vi "WriteLog.vi"(8 "error in (no error)":errorcluster, 10 "Loop Counter":i32, 11 "Channel Manager in":refnum<class "Channel Manager.lvclass">) -> (0 "error out":errorcluster, 3 "Channel Manager out":refnum<class "Channel Manager.lvclass">)   [LabVIEW 2024, in "Embedded TDMS Logger Engine.lvlib" / "Channel Manager.lvclass"]
doc: "Write to our TDMS file if the trigger is active."
uses:
  Channel Manager.lvclass
  Channel Manager.lvclass/Channel Manager.ctl
  Shared/File Classes/File/File.lvclass
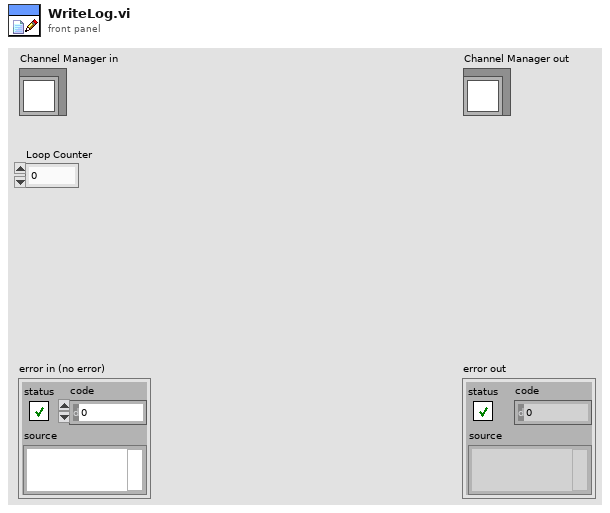
[diagram p1: front panel]
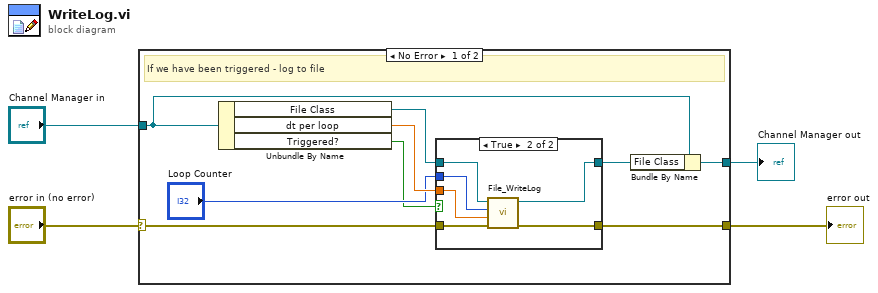
[diagram p0: block diagram]
diagram:
  n1 = case shown="No Error" "error in (no error)" {
    selector: "error in (no error)" -> [w10 w23]
    tunnel: [w9 w23] -> w3
    tunnel: [w7 w22] -> w1
    tunnel: "Channel Manager in" -> [w8 w22]
    frame No Error {
      # "If we have been triggered - log to file"
      n2 = Unbundle By Name(w8) -> ("File Class"=w13:refnum<class "File.lvclass">, "dt per loop"=w12:dbl, "Triggered?"=w5:bool)
      n3 = case shown="True" w5 {
        tunnel: w13 -> [w15 w21]
        tunnel: w12 -> [_ w20]
        tunnel: "Loop Counter" -> [_ w19]
        tunnel: w10 -> [w14 w16]
        tunnel: [w14 w18] -> w9
        tunnel: [w15 w17] -> w6
        frame False {
        }
        frame True {
          n4 = call-dynamic "File_WriteLog.vi"("error in (no error)"=w16, "dt per loop"=w20, "Loop Counter"=w19, "File in"=w21) -> ("error out"=w18:errorcluster, "File out"=w17:refnum<class "File.lvclass">)  [unwired: 6 in]
        }
      }
      n5 = Bundle By Name(cluster=w8, "File Class"=w6) -> (w7:refnum<class "Channel Manager.lvclass">)
    }
    frame Error {
    }
  }
  "error out" <- w3
  "Channel Manager out" <- w1
